vi "Dequeue.vi"(8 "ErrorArray":errorcluster[](array[cluster])) -> (0 "ErrorArray":errorcluster[](array[cluster]), 1 "Message Data":variant, 2 "Message":string)   [LabVIEW 2014, in "Queue.lvlib"]
uses:
  Queue.lvlib
  <userlib>/NIST/NISTErrorLib/NISTErrorLib.lvlib
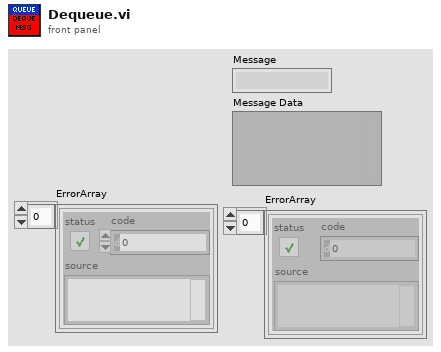
[diagram p1: front panel]
types:
  T1 = typedef "Queue.lvlib/clMessage.ctl" = cluster{"Message":string, "Message Data":variant}
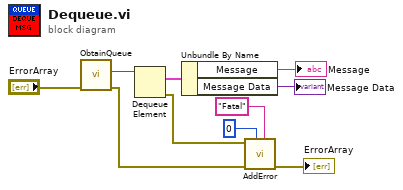
[diagram p0: block diagram]
diagram:
  n1 = call "ObtainQueue.vi"("ErrorArray"="ErrorArray") -> ("ErrorArray"=w5:errorcluster[], "QueueRef"=w7:refnum<queue>)  [unwired: 9 in]
  n2 = Dequeue Element(queue=w7) -> (element=w10:T1, error out=w4:errorcluster)  [unwired: 2 in, 2 out]
  n3 = Unbundle By Name(w10) -> ("Message"=→"Message":string, "Message Data"=→"Message Data":variant)
  n4 = call <userlib>:"AddError.vi"("Severity"="Fatal", "Priority"=u8 0, "ErrorArray"=w5, "error in (no error)"=w4) -> ("ErrorArray"=→"ErrorArray":errorcluster[])  [unwired: 6 in, 1 out]
